vi "Calibration Equipment.vi"() -> ()   [LabVIEW 2018]
uses:
  Type Definitions/Calibration Time.ctl
  Type Definitions/Calibration SN.ctl
  Type Definitions/Calibration.ctl
panel:
  in  "Complete":bool
  in  "Calibration ID":T1
  in  "SN":T2
  in  "Calibration\nDue Date":T3 {"Eq20" format="%<%x>T"; "Eq19" format="%<%x>T"; "Eq18" format="%<%x>T"; "Eq17" format="%<%x>T"; "Eq16" format="%<%x>T"; "Eq15" format="%<%x>T"; "Eq14" format="%<%x>T"; "Eq13" format="%<%x>T"; "Eq12" format="%<%x>T"; "Eq11" format="%<%x>T"; "Eq10" format="%<%x>T"; "Eq9" format="%<%x>T"; "Eq8" format="%<%x>T"; "Eq7" format="%<%x>T"; "Eq6" format="%<%x>T"; "Eq5" format="%<%x>T"; "Eq4" format="%<%x>T"; "Eq3" format="%<%x>T"; "Eq2" format="%<%x>T"; "Eq1" format="%<%x>T"}
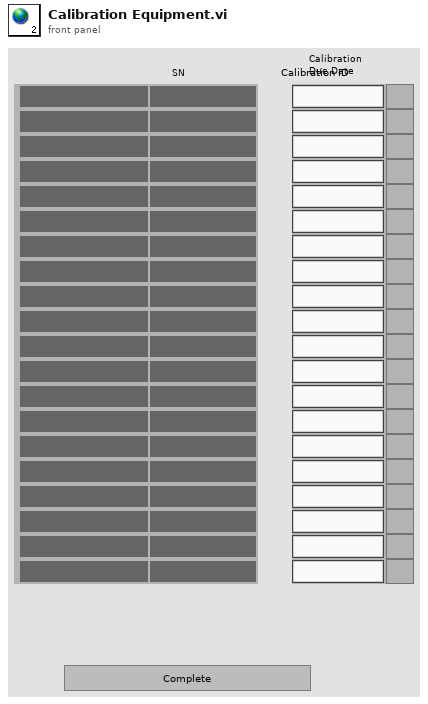
[diagram p1: front panel]
types:
  T1 = typedef "Calibration.ctl" = cluster{"Eq 1":string, "Eq 2":string, "Eq 3":string, "Eq 4":string, "Eq 5":string, "Eq 6":string, "Eq 7":string, "Eq 8":string, "Eq 9":string, "Eq 10":string, "Eq 11":string, "Eq 12":string, "Eq 13":string, "Eq 14":string, "Eq 15":string, "Eq 16":string, "Eq 17":string, "Eq 18":string, "Eq 19":string, "Eq 20":string}
  T2 = typedef "Calibration SN.ctl" = cluster{"Eq 1":string, "Eq 2":string, "Eq 3":string, "Eq 4":string, "Eq 5":string, "Eq 6":string, "Eq 7":string, "Eq 8":string, "Eq 9":string, "Eq 10":string, "Eq 11":string, "Eq 12":string, "Eq 13":string, "Eq 14":string, "Eq 15":string, "Eq 16":string, "Eq 17":string, "Eq 18":string, "Eq 19":string, "Eq 20":string}
  T3 = typedef "Calibration Time.ctl" = cluster{"Eq1":timestamp, "Eq2":timestamp, "Eq3":timestamp, "Eq4":timestamp, "Eq5":timestamp, "Eq6":timestamp, "Eq7":timestamp, "Eq8":timestamp, "Eq9":timestamp, "Eq10":timestamp, "Eq11":timestamp, "Eq12":timestamp, "Eq13":timestamp, "Eq14":timestamp, "Eq15":timestamp, "Eq16":timestamp, "Eq17":timestamp, "Eq18":timestamp, "Eq19":timestamp, "Eq20":timestamp}
diagram:
